vi "SP - set value array STR.vi"(8 "error in (no error)":errorcluster, 11 "JSON string":string) -> (0 "error out":errorcluster, 3 "value":string)   [LabVIEW 2020, in "ui-testing.lvlib"]
doc: "copyright: Thomas Zilliox©"
uses:
  ui-testing.lvlib
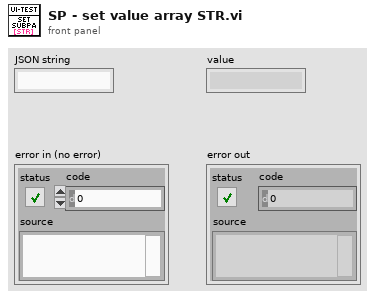
[diagram p1: front panel]
types:
  T1 = cluster{"subpanel":string, "control":string, "value":string[]}
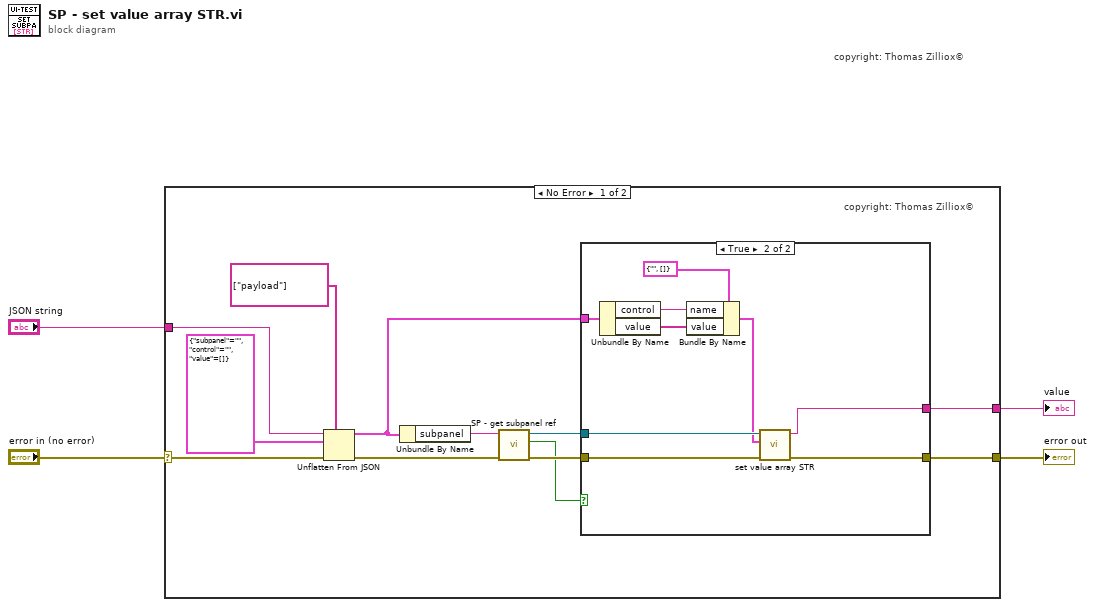
[diagram p0: block diagram]
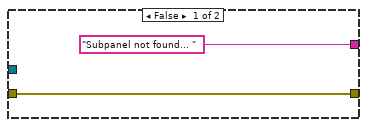
[diagram p2: hidden frame]
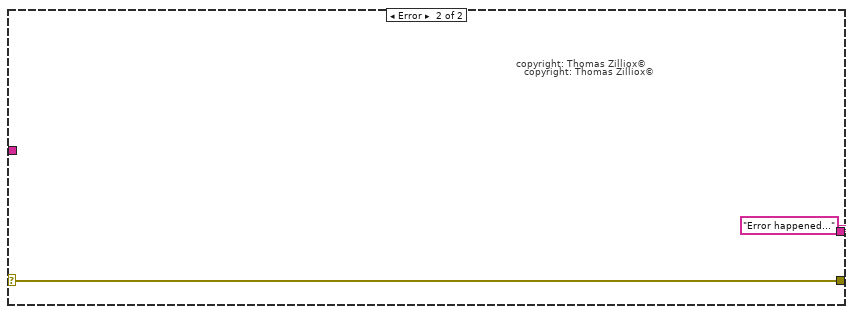
[diagram p3: hidden frame]
diagram:
  # "copyright: Thomas Zilliox©"
  n1 = case shown="No Error" "error in (no error)" {
    selector: "error in (no error)" -> [w12 w29]
    tunnel: "JSON string" -> [w14 _]
    tunnel: [w13 w29] -> w3
    tunnel: [w10 "Error happened..."] -> w1
    frame No Error {
      # "copyright: Thomas Zilliox©"
      n2 = Unflatten From JSON(path=string[] ["payload"], JSON string=w14, type and defaults=T1 {"subpanel"="", "control"="", "value"=[]}, error in (no error)=w12) -> (value=w9:T1, error out=w15:errorcluster)  [unwired: 3 in]
      n3 = Unbundle By Name(w9) -> ("subpanel"=w8:string)
      n4 = call "SP - get subpanel ref.vi"("error in (no error)"=w15, "subpanel"=w8) -> ("error out"=w6:errorcluster, "subpanel found ?"=w5:bool, "subpanel ref"=w7:refnum<vi>)  [unwired: 7 in]
      n5 = case shown="True" w5 {
        tunnel: [w18 w25] -> w13
        tunnel: w7 -> [_ w27]
        tunnel: w6 -> [w18 w24]
        tunnel: ["Subpanel not found... " ("result string") w26] -> w10
        tunnel: w9 -> [_ w21]
        frame False {
        }
        frame True {
          n6 = Unbundle By Name(w21) -> ("control"=w19:string, "value"=w20:string[])
          n7 = Bundle By Name(cluster=cluster{"name":string, "value":string[]} {"name"="", "value"=[]} ("Payload"), "name"=w19, "value"=w20) -> (w22:cluster{"name":string, "value":string[]})
          n8 = call "set value array STR.vi"("error in (no error)"=w24, "Payload"=w22, "VI Ref"=w27) -> ("error out"=w25:errorcluster, "return value"=w26:string)  [unwired: 7 in]
        }
      }
    }
    frame Error {
      # "copyright: Thomas Zilliox©"
      # "copyright: Thomas Zilliox©"
    }
  }
  "error out" <- w3
  "value" <- w1
